vi "CMI LiB Bias Read Error.vi"(8 "error in":errorcluster, 11 "VISA in":refnum<visa-resource-name>) -> (0 "error out":errorcluster, 2 "error string":string, 3 "VISA out":refnum<visa-resource-name>)   [LabVIEW 2013]
uses:
  <vilib>/ErrorRing/Error Ring.xnode
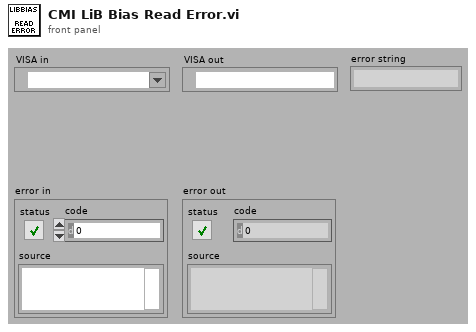
[diagram p1: front panel]
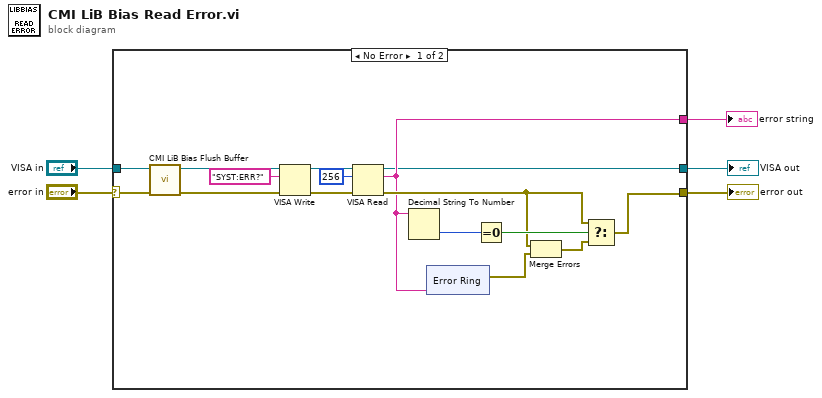
[diagram p0: block diagram]
diagram:
  n1 = case shown="No Error" "error in" {
    selector: "error in" -> [w9 w28]
    tunnel: "VISA in" -> [w8 w27]
    tunnel: [w10 w27] -> w4
    tunnel: [w12 w28] -> w3
    tunnel: [w11 _] -> w2
    frame No Error {
      n2 = call "CMI LiB Bias Flush Buffer.vi"("error in"=w9, "VISA in"=w8) -> ("error out"=w6:errorcluster, "VISA out"=w7:refnum<visa-resource-name>)  [unwired: 8 in]
      n3 = VISA Write(VISA resource name=w7, write buffer="SYST:ERR?", error in (no error)=w6) -> (VISA resource name out=w19:refnum<visa-resource-name>, error out=w20:errorcluster)  [unwired: 1 out]
      n4 = VISA Read(VISA resource name=w19, byte count=u32 256, error in (no error)=w20) -> (VISA resource name out=w10:refnum<visa-resource-name>, read buffer=w11:string, error out=w14:errorcluster)  [unwired: 1 out]
      n5 = Decimal String To Number(string=w11) -> (number=w17:i32)  [unwired: 2 in, 1 out]
      n6 = xnode "Error Ring"("parameter 0"=w11) -> ("error out"=w13:errorcluster)
      n7 = Equal To 0?(x=w17) -> (x = 0?=w16:bool)
      n8 = Merge Errors(w14, w13) -> (w15:errorcluster)
      n9 = Select(t=w14, s=w16, f=w15) -> (s? t:f=w12:errorcluster)
    }
    frame Error {
    }
  }
  "error out" <- w3
  "VISA out" <- w4
  "error string" <- w2
